vi "Rational Resample (single channel, DBL).vi"(5 "anti-aliasing?":bool=TRUE, 6 "FIR filter specifications":T1={"alias rejection (dB)"=120.0, "normalized bandwidth"=0.4536} {"normalized bandwidth" format="%.4f"; "alias rejection (dB)" format="%.2f"}, 7 "reset":bool, 8 "error in (no error)":errorcluster, 9 "resample factor":cluster{"interpolation":i32, "decimation":i32}={"interpolation"=1, "decimation"=1}, 10 "start index":i32, 11 "X":dbl[](array[numeric])) -> (0 "error out":errorcluster, 2 "t0":dbl, 3 "Y":dbl[](array[numeric]))   [LabVIEW 2017, in "NI_AALPro.lvlib"]
doc: "Resamples the input signal <B>X</B> by interpolating <B>X</B>, passing the interpolated signal through an FIR filter, and decimating the filtered signal. Wire data to the <B>X</B> input to determine the polymorphic instance to use or manually select the instance."
uses:
  NI_AALPro.lvlib
  <resource>/lvanlys.dll
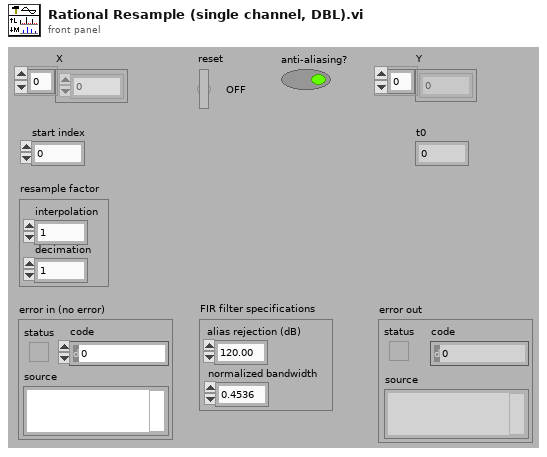
[diagram p1: front panel]
types:
  T1 = cluster{"alias rejection (dB)":dbl, "normalized bandwidth":dbl}
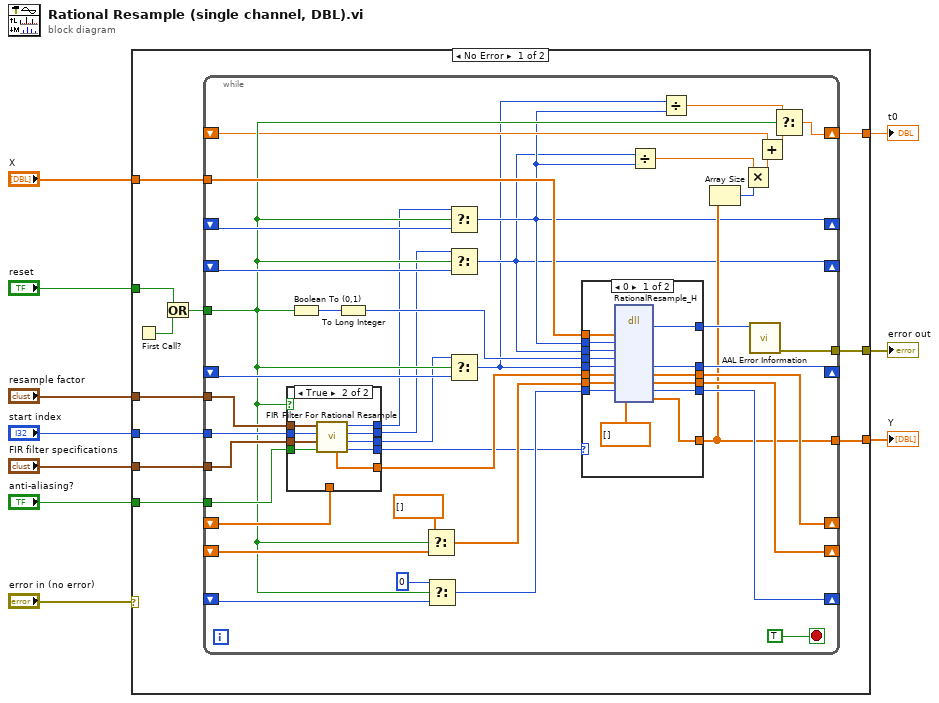
[diagram p0: block diagram]
diagram:
  n1 = case shown="No Error" "error in (no error)" {
    selector: "error in (no error)" -> [_ w89]
    tunnel: "X" -> [w21 _]
    tunnel: "FIR filter specifications" -> [w20 _]
    tunnel: "start index" -> [w19 _]
    tunnel: [w18 w89] -> w7
    tunnel: "resample factor" -> [w17 _]
    tunnel: [w16 _] -> w5
    tunnel: "anti-aliasing?" -> [w15 _]
    tunnel: [w14 _] -> w2
    tunnel: "reset" -> [w11 _]
    frame No Error {
      n2 = First Call?() -> (First Call?: T/F=w13:bool)
      n3 = Or(x=w11, y=w13) -> (x .or. y?=w12:bool)
      n4 = while {
        tunnel: w21 -> [w62]
        shift-right: [w25] -> _
        shift-left: _ -> [w60]
        tunnel: w12 -> [w36]
        shift-right: [w24] -> _
        shift-left: _ -> [w59]
        shift-right: [w42] -> _
        shift-left: _ -> [w56]
        shift-right: [w43] -> _
        shift-left: _ -> [w54]
        shift-right: [w49] -> _
        shift-left: _ -> [w50]
        shift-right: [w46] -> _
        shift-left: _ -> [w45]
        tunnel: w20 -> [w48]
        tunnel: w19 -> [w44]
        tunnel: [w40] -> w18
        tunnel: w17 -> [w39]
        tunnel: [w33] -> w16
        tunnel: w15 -> [w37]
        shift-right: [w34] -> w14
        shift-left: _ -> [w32]
        stop <- TRUE stop-if-true
        n5 = case shown="True" w36 {
          tunnel: [w79 w82] -> w47
          tunnel: w48 -> [_ w83]
          tunnel: w45 -> [w79 _]
          tunnel: [_ w88] -> w30
          tunnel: [_ w87] -> w31
          tunnel: w44 -> [_ w84]
          tunnel: [_ w86] -> w22
          tunnel: w39 -> [_ w85]
          tunnel: [_ w81] -> w38
          tunnel: w37 -> [_ w80]
          frame False {
          }
          frame True {
            n6 = call "FIR Filter For Rational Resample.vi"("anti-aliasing?"=w80, "FIR filter specifications"=w83, "start index"=w84, "resample factor"=w85) -> ("error"=w81:i32, "start index out"=w86:i32, "decimation"=w87:i32, "interpolation out"=w88:i32, "filter coefficients"=w82:dbl[])  [unwired: 3 in]
          }
        }
        n7 = Boolean To (0,1)(Boolean=w36) -> (0, 1=w58:i16)
        n8 = To Long Integer(number=w58) -> (32bit integer=w57:i32)
        n9 = Select(t=dbl[] [] ("yH"), s=w36, f=w56) -> (s? t:f=w52:dbl[])
        n10 = Select(t=0, s=w36, f=w54) -> (s? t:f=w53:i32)
        n11 = Select(t=w30, s=w36, f=w60) -> (s? t:f=w25:i32)
        n12 = Select(t=w31, s=w36, f=w59) -> (s? t:f=w24:i32)
        n13 = Select(t=w22, s=w36, f=w50) -> (s? t:f=w23:i32)
        n14 = case shown="0" w38 {
          selector: w38 -> [_ w78]
          tunnel: w62 -> [w77 _]
          tunnel: w25 -> [w76 _]
          tunnel: w24 -> [w75 _]
          tunnel: w57 -> [w74 _]
          tunnel: w53 -> [w73 _]
          tunnel: w52 -> [w72 _]
          tunnel: w23 -> [w71 _]
          tunnel: [w70 _] -> w49
          tunnel: w47 -> [w69 _]
          tunnel: [w68 _] -> w46
          tunnel: [w67 _] -> w43
          tunnel: [w66 _] -> w42
          tunnel: [w65 w78] -> w41
          tunnel: [w64 _] -> w33
          frame 0 {
            n15 = dll-call lib="C:/Program Files (x86)/National Instruments/LabVIEW 2017/resource/lvanlys.*" fn="RationalResample_H"("X"=w77, "interpolation"=w76, "decimation"=w75, "reset"=w74, "startIndex"=w71, "filterH"=w69, "bufferH"=w72, "singalSizeInBuffer"=w73, "yH"=dbl[] []) -> (w65:i32, "startIndex"=w70:i32, "filterH"=w68:dbl[], "bufferH"=w66:dbl[], "singalSizeInBuffer"=w67:i32, "yH"=w64:dbl[])  [unwired: 7 in, 2 out]
          }
          frame 1, Default {
          }
        }
        n16 = Divide(x=w24, y=w25) -> (x/y=w28:dbl)
        n17 = Divide(x=w23, y=w25) -> (x/y=w35:dbl)
        n18 = Array Size(array=w33) -> (size(s)=w29:i32)
        n19 = Multiply(x=w28, y=w29) -> (x*y=w27:dbl)
        n20 = call "AAL Error Information.vi"("error code"=w41) -> ("error out"=w40:errorcluster)  [unwired: 10 in]
        n21 = Add(x=w32, y=w27) -> (x+y=w26:dbl)
        n22 = Select(t=w35, s=w36, f=w26) -> (s? t:f=w34:dbl)
      }
    }
    frame Error {
    }
  }
  "error out" <- w7
  "Y" <- w5
  "t0" <- w2
